vi "loop2.vi"() -> ()   [LabVIEW 2013]
uses:
  globalcontrols.vi
panel:
  out "Loop 2 Light":bool
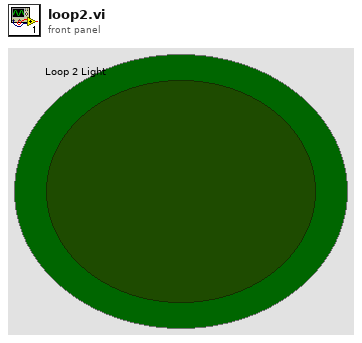
[diagram p1: front panel]
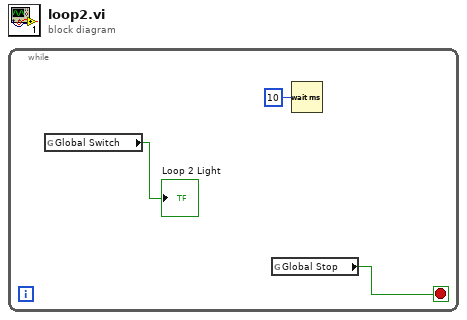
[diagram p0: block diagram]
diagram:
  n1 = while {
    stop <- w2 stop-if-true
    n2 = global read "globalcontrols.vi" "Global Switch"() -> (→"Loop 2 Light":bool)
    n3 = global read "globalcontrols.vi" "Global Stop"() -> (w2:bool)
    n4 = Wait (ms)(milliseconds to wait=u32 10) -> ()  [unwired: 1 out]
  }
